vi "Test 4 X Coordinate of Crosspoint.vi"(8 "error in (no error)":errorcluster, 11 "Test Case In":refnum<class "Vector Test.lvclass">) -> (0 "error out":errorcluster, 3 "Test Case Out":refnum<class "Vector Test.lvclass">)   [LabVIEW 2021, in "Vector Test.lvclass"]
uses:
  Vector Test.lvclass
  C:/Program Files (x86)/National Instruments/LabVIEW 2021/vi.lib/Astemes/LUnit/Test Case.lvclass
  <vilib>/Astemes/LUnit/Test Case.lvclass/Test Case.ctl
  5eaabc76-4b9d-4a93-b043-85ec81865f2e.vi
  <vilib>/Astemes/LUnit/Append Pass Result.vi
  <vilib>/Astemes/LUnit/Append Fail Result.vi
  <vilib>/Astemes/LUnit/Describe Comparison.vi
  <vilib>/Astemes/LUnit/Compare Variants.vi
  <vilib>/Astemes/LUnit/Variant to string.vi
  <vilib>/Utility/Data Type/Get Type Information.vi
  <vilib>/Utility/LVClass/Get LV Class Name.vi
  Vector/Vector.lvclass
  High Res Arithmetic/Rational Number.lvclass
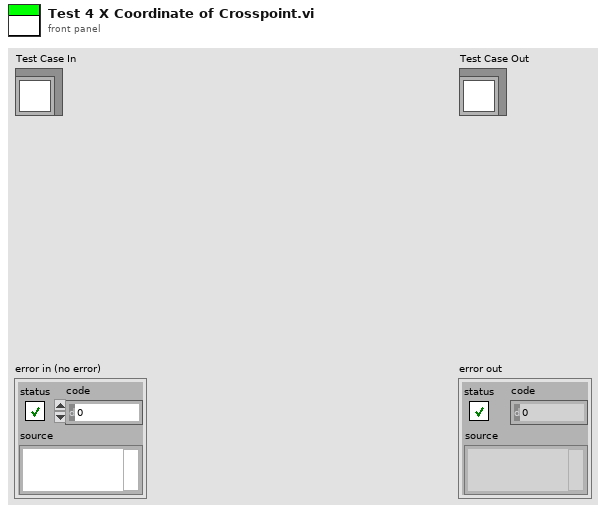
[diagram p1: front panel]
types:
  T1 = cluster{"X":refnum<class "Rational Number.lvclass">, "Y":refnum<class "Rational Number.lvclass">}
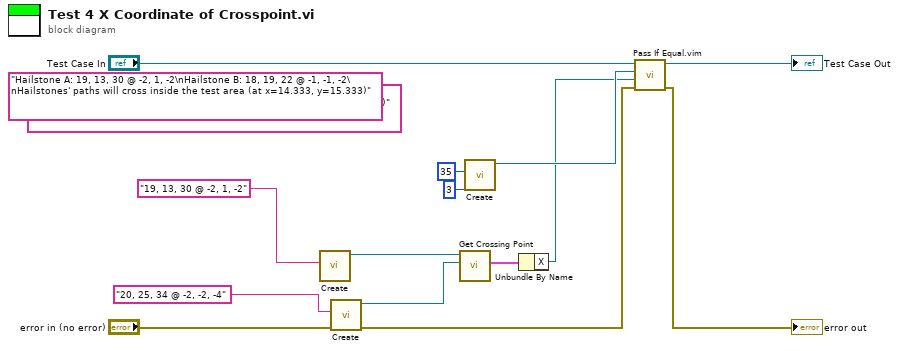
[diagram p0: block diagram]
diagram:
  (unwired) "Hailstone A: 19, 13, 30 @ -2, 1, -2\nHailstone B: 20, 25, 34 @ -2, -2, -4\nHailstones' paths will cross inside the test area (at x=11.667, y=16.667)" ("Input")
  (unwired) "Hailstone A: 19, 13, 30 @ -2, 1, -2\nHailstone B: 18, 19, 22 @ -1, -1, -2\nHailstones' paths will cross inside the test area (at x=14.333, y=15.333)" ("Input")
  n1 = call "Create.vi"("Input"="19, 13, 30 @ -2, 1, -2") -> ("Hailstone Out"=w7:refnum<class "Vector.lvclass">)  [unwired: 9 in, 1 out]
  n2 = call "Create.vi"("error in (no error)"="error in (no error)", "Input"="20, 25, 34 @ -2, -2, -4") -> ("error out"=w10:errorcluster, "Hailstone Out"=w6:refnum<class "Vector.lvclass">)  [unwired: 8 in]
  n3 = call "Get Crossing Point.vi"("Vector 2"=w6, "Vector in"=w7) -> ("Coordinate"=w2:T1)  [unwired: 8 in, 1 out]
  n4 = call "Create.vi"("Denumerator"=i64 3, "Numerator"=i64 35) -> ("Hi Res Arithm Test"=w3:refnum<class "Rational Number.lvclass">)  [unwired: 8 in, 1 out]
  n5 = Unbundle By Name(w2) -> ("X"=w1:refnum<class "Rational Number.lvclass">)
  n6 = call "Pass If Equal.vim"("error in (no error)"=w10, "Actual"=w1, "Expected"=w3, "LUnit Test Case In"="Test Case In") -> ("error out"=→"error out":errorcluster, "LUnit Test Case Out"=→"Test Case Out":refnum<class "Vector Test.lvclass">)  [unwired: 6 in]
